vi "Video Select Source.vi"(1 "Cluster In":T3, 2 "Source Name":string, 3 "Bool Refnum":refnum<vi>) -> (0 "Cluster Out":T3)   [LabVIEW 2010]
uses:
  System.Windows.Forms
  drivers/DirectShow SDK/v10/DirectShow SDK.llb/DirectShow - Capture Device.ctl
  D:/Projekte/Promotion/Scripts/LabView/drivers/DirectShow SDK/lib/DirectShowLib-2005.dll
  drivers/DirectShow SDK/lib/DirectShowLib-2005.dll
  drivers/DirectShow SDK/v10/DirectShow SDK.llb/DirectShow - Media State.ctl
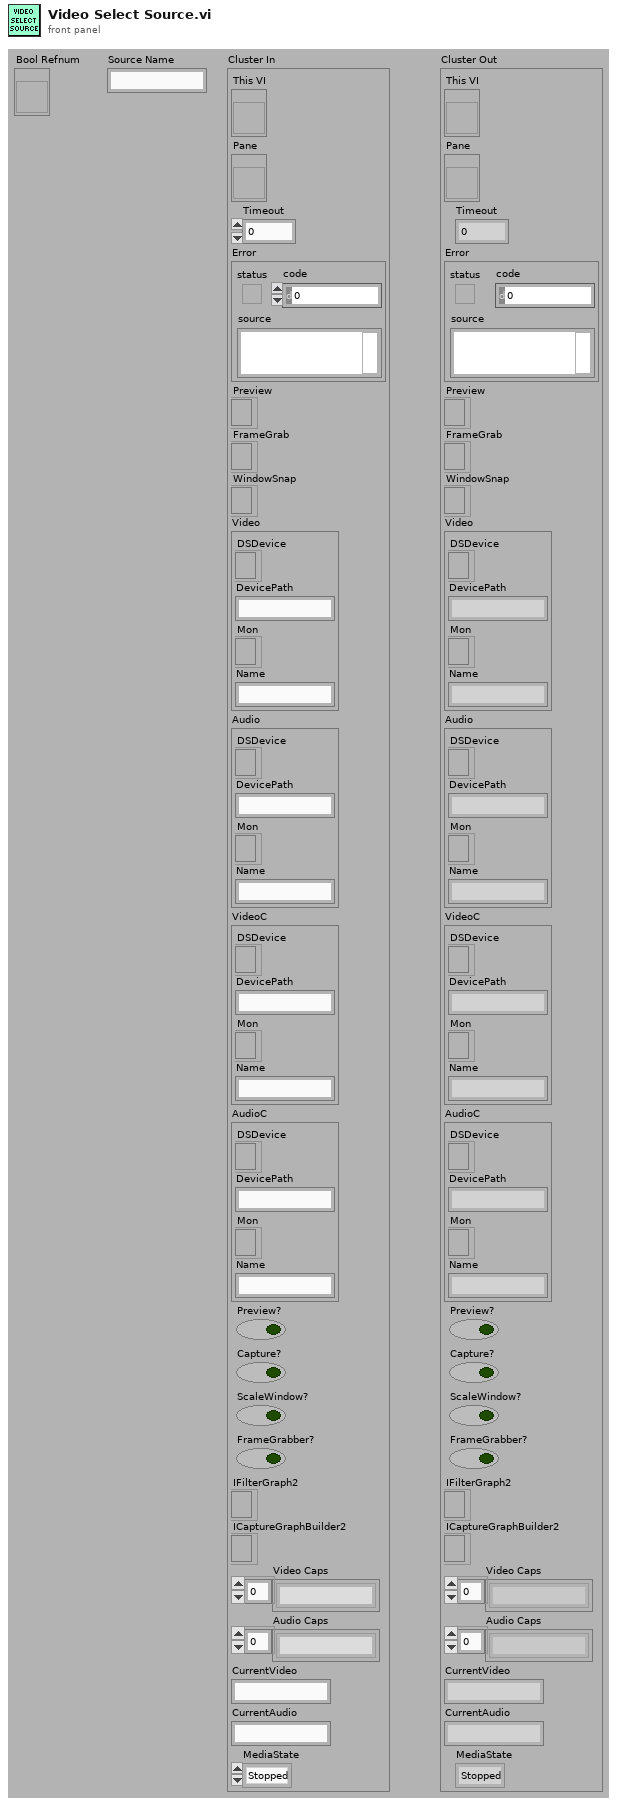
[diagram p1: front panel]
types:
  T1 = typedef "DirectShow - Capture Device.ctl" = cluster{"DSDevice":refnum<k24>, "DevicePath":string, "Mon":refnum<k24>, "Name":string}
  T2 = typedef "DirectShow - Media State.ctl" = enum16{"Stopped", "Playing", "Paused", "Recording"}
  T3 = cluster{"This VI":refnum<vi>, "Pane":refnum<vi>, "Timeout":i32, "Error":errorcluster, "Preview":refnum<k24>, "FrameGrab":refnum<k24>, "WindowSnap":refnum<k24>, "Video":T1, "Audio":T1, "VideoC":T1, "AudioC":T1, "Preview?":bool, "Capture?":bool, "ScaleWindow?":bool, "FrameGrabber?":bool, "IFilterGraph2":refnum<k24>, "ICaptureGraphBuilder2":refnum<k24>, "Video Caps":string[], "Audio Caps":string[], "CurrentVideo":string, "CurrentAudio":string, "MediaState":T2}
  T4 = enum8{"Enabled", "Disabled", "Disabled and Grayed Out"}
  T5 = enum16{"AnalogVideoIn", "Capture", "CC", "EDS", "NABTS", "Preview", "Still", "TeleText", "TimeCode", "VBI", "VideoPort", "VideoPortVBI"}
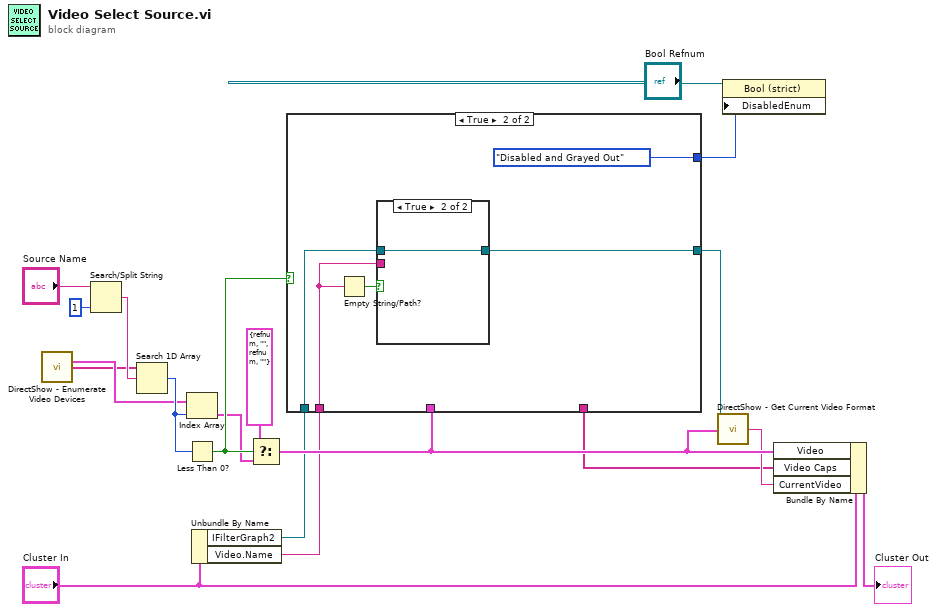
[diagram p0: block diagram]
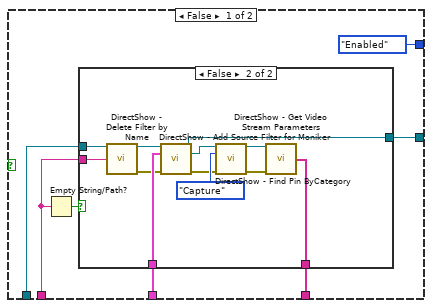
[diagram p2: hidden frame]
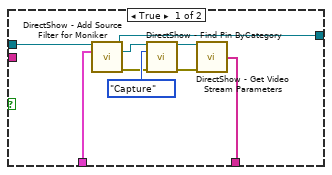
[diagram p3: hidden frame]
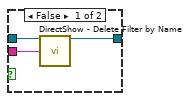
[diagram p4: hidden frame]
diagram:
  n1 = call "DirectShow - Enumerate Video Devices.vi"() -> ("Devices"=w6:T1[], "Names"=w4:string[])  [unwired: 13 in, 1 out]
  n2 = Search/Split String(string="Source Name", offset (0)=1) -> (match + rest of string=w5:string)  [unwired: 1 in, 2 out]
  n3 = Search 1D Array(1D array=w4, element=w5) -> (index of element=w8:i32)  [unwired: 1 in]
  n4 = Index Array(array=w6, index=w8) -> (element=w9:T1)
  n5 = Less Than 0?(x=w8) -> (x < 0?=w11:bool)
  n6 = Unbundle By Name("Cluster In") -> ("IFilterGraph2"=w14:refnum<k24>, "Video.Name"=w15:string)
  n7 = Select(t=T1 {"DSDevice"=refnum, "DevicePath"="", "Mon"=refnum, "Name"=""}, s=w11, f=w9) -> (s? t:f=w18:T1)
  n8 = case shown="True" w11 {
    tunnel: [w26 _] -> w12
    tunnel: w14 -> [w25 w52]
    tunnel: w15 -> [w22 w51]
    tunnel: w18 -> [w23 _]
    tunnel: [w21 w49] -> w16
    tunnel: [T4."Enabled" ("Disabled") T4."Disabled and Grayed Out" ("Disabled")] -> w19
    frame False {
      n9 = Empty String/Path?(string/path=w22) -> (empty?=w24:bool)
      n10 = case shown="False" w24 {
        tunnel: [w27 w36] -> w26
        tunnel: w25 -> [w30 w41]
        tunnel: w23 -> [w29 w42]
        tunnel: w22 -> [_ w38]
        tunnel: [w28 w37] -> w21
        frame True {
          n11 = call "DirectShow - Add Source Filter for Moniker.vi"("IFilterGraph2"=w30, "Device"=w29) -> ("IFilterGraph2 dup"=w28:refnum<k24>, "ppFilter"=w33:refnum<k24>, "error out"=w34:errorcluster)  [unwired: 11 in]
          n12 = call "DirectShow - Find Pin ByCategory.vi"("Source"=w33, "Category"=T5."Capture", "error in (no error)"=w34) -> ("DS_Pin"=w32:refnum<k24>, "error out"=w31:errorcluster)  [unwired: 11 in]
          n13 = call "DirectShow - Get Video Stream Parameters.vi"("Stream"=w32, "error in (no error)"=w31) -> ("Abbreviated"=w27:string[])  [unwired: 9 in, 4 out]
        }
        frame False {
          n14 = call "DirectShow - Delete Filter by Name.vi"("IFilterGraph2"=w41, "pName"=w38) -> ("IFilterGraph2 dup"=w40:refnum<k24>, "error out"=w39:errorcluster)  [unwired: 12 in]
          n15 = call "DirectShow - Add Source Filter for Moniker.vi"("IFilterGraph2"=w40, "Device"=w42, "error in (no error)"=w39) -> ("IFilterGraph2 dup"=w37:refnum<k24>, "ppFilter"=w45:refnum<k24>, "error out"=w46:errorcluster)  [unwired: 10 in]
          n16 = call "DirectShow - Find Pin ByCategory.vi"("Source"=w45, "Category"=T5."Capture", "error in (no error)"=w46) -> ("DS_Pin"=w44:refnum<k24>, "error out"=w43:errorcluster)  [unwired: 11 in]
          n17 = call "DirectShow - Get Video Stream Parameters.vi"("Stream"=w44, "error in (no error)"=w43) -> ("Abbreviated"=w36:string[])  [unwired: 9 in, 4 out]
        }
      }
    }
    frame True {
      n18 = Empty String/Path?(string/path=w51) -> (empty?=w50:bool)
      n19 = case shown="True" w50 {
        tunnel: w52 -> [w55 w56]
        tunnel: w51 -> [w54 _]
        tunnel: [w53 w56] -> w49
        frame False {
          n20 = call "DirectShow - Delete Filter by Name.vi"("IFilterGraph2"=w55, "pName"=w54) -> ("IFilterGraph2 dup"=w53:refnum<k24>)  [unwired: 12 in, 1 out]
        }
        frame True {
        }
      }
    }
  }
  n21 = call "DirectShow - Get Current Video Format.vi"("IFilterGraph2"=w16, "Video"=w18) -> ("Abbreviated"=w17:string)  [unwired: 10 in, 3 out]
  n22 = property on="Property Node" class="Bool (strict)"(reference="Bool Refnum", "DisabledEnum"=w19) -> ()  [unwired: 1 in, 2 out]
  n23 = Bundle By Name(cluster="Cluster In", "Video"=w18, "Video Caps"=w12, "CurrentVideo"=w17) -> (→"Cluster Out":T3)
